vi "refresh.vi"(8 "error in (no error)":errorcluster, 10 "Engine Configuration In":refnum<class "engine configuration.lvclass">, 11 "tag bus configurable plugin editor node In":refnum<class "tag bus configurable plugin editor node.lvclass">) -> (0 "error out":errorcluster, 2 "Engine Configuration Out":refnum<class "engine configuration.lvclass">, 3 "tag bus configurable plugin editor node Out":refnum<class "tag bus configurable plugin editor node.lvclass">)   [LabVIEW 2013, in "tag bus configurable plugin editor node.lvclass"]
uses:
  tag bus configurable plugin editor node.lvclass
  <vilib>/NI/Module Execution Interface/Engine Configuration/engine configuration.lvclass
  <vilib>/NI/Tag Bus Data Framework/Configuration Editor/Classes/Module editor node/module editor node.lvclass
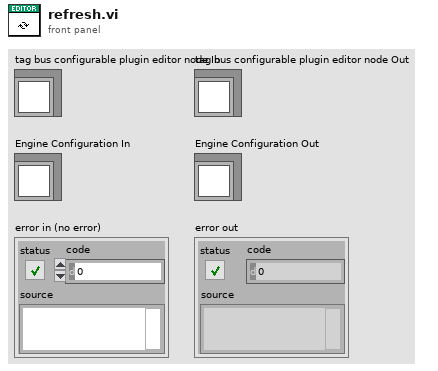
[diagram p1: front panel]
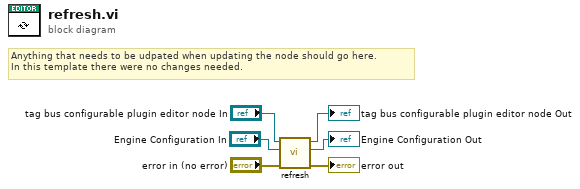
[diagram p0: block diagram]
diagram:
  # "Anything that needs to be udpated when updating the node should go here.\nIn this template there were no changes needed."
  n1 = call-parent "refresh.vi"("error in (no error)"="error in (no error)", "Engine Configuration In"="Engine Configuration In", "Module Editor Node In"="tag bus configurable plugin editor node In") -> ("error out"=→"error out":errorcluster, "Engine Configuration Out"=→"Engine Configuration Out":refnum<class "engine configuration.lvclass">, "Module Editor Node Out"=→"tag bus configurable plugin editor node Out":refnum<class "tag bus configurable plugin editor node.lvclass">)  [unwired: 6 in]
